vi "RECIPE_NAME_DOWNLOAD.vi"(8 "error in (no error)":errorcluster, 9 "Recipe Names":string[][](array[string]), 10 "appended array":refnum<vi>[](array[refnum])) -> (0 "error out":errorcluster)   [LabVIEW 2017]
panel:
  in  "PRODUCT LIST":string(combo)
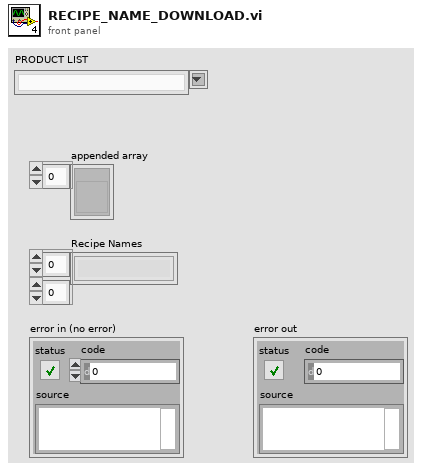
[diagram p1: front panel]
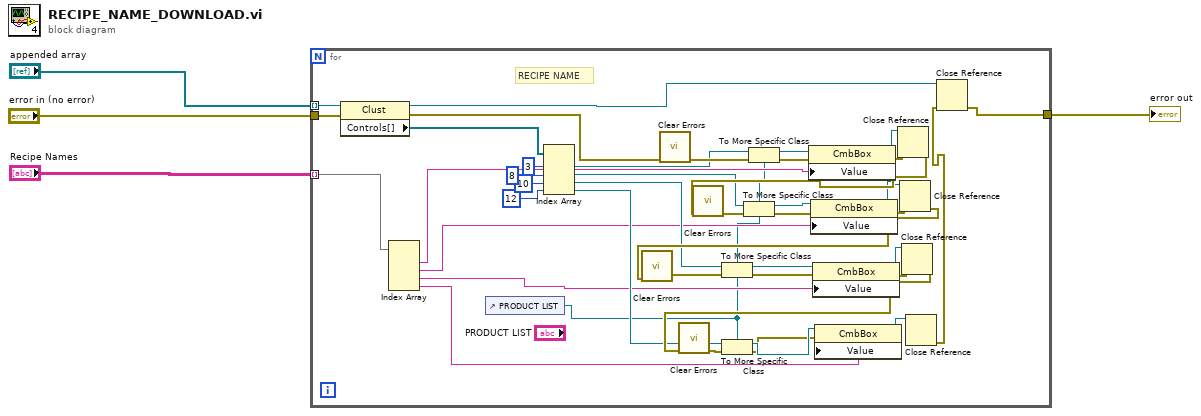
[diagram p0: block diagram]
diagram:
  n1 = for {
    tunnel: [w44] -> w1
    tunnel: "appended array" -> [w47] mode=indexing
    tunnel: "error in (no error)" -> [w46]
    tunnel: "Recipe Names" -> [w27] mode=indexing
    # "RECIPE NAME"
    n2 = property class="Clust"(reference=w47, error in=w46) -> (reference out=w43:refnum<vi>, error out=w45:errorcluster, "Controls[]"=w41:refnum<vi>[])
    n3 = Index Array(array=w27) -> (element #1=w23:string, element #2=w8:string, element #3=w7:string, element #4=w6:string)  [unwired: 4 in]
    n4 = control-ref of="PRODUCT LIST"() -> (w5:refnum<vi>)
    n5 = Index Array(array=w41, index #1=3 ("index"), index #2=8 ("index"), index #3=10 ("index"), index #4=12 ("index")) -> (element #1=w9:refnum<vi>, element #2=w13:refnum<vi>, element #3=w18:refnum<vi>, element #4=w26:refnum<vi>)
    n6 = call <vilib>:"Clear Errors.vi"("error in (no error)"=w45) -> ("error out"=w12:errorcluster)  [unwired: 5 in, 1 out]
    n7 = To More Specific Class(target class=w5, reference=w9, error in=w12) -> (specific class reference=w10:refnum<vi>, error out=w11:errorcluster)
    n8 = property class="CmbBox"(reference=w10, error in=w11, "Value"=w23) -> (reference out=w30:refnum<vi>, error out=w42:errorcluster)
    n9 = Close Reference(reference=w30, error in (no error)=w42) -> (error out=w33:errorcluster)
    n10 = call <vilib>:"Clear Errors.vi"("error in (no error)"=w33) -> ("error out"=w16:errorcluster)  [unwired: 5 in, 1 out]
    n11 = To More Specific Class(target class=w5, reference=w13, error in=w16) -> (specific class reference=w14:refnum<vi>, error out=w15:errorcluster)
    n12 = property class="CmbBox"(reference=w14, error in=w15, "Value"=w8) -> (reference out=w29:refnum<vi>, error out=w36:errorcluster)
    n13 = Close Reference(reference=w29, error in (no error)=w36) -> (error out=w32:errorcluster)
    n14 = call <vilib>:"Clear Errors.vi"("error in (no error)"=w32) -> ("error out"=w19:errorcluster)  [unwired: 5 in, 1 out]
    n15 = To More Specific Class(target class=w5, reference=w18, error in=w19) -> (specific class reference=w17:refnum<vi>, error out=w20:errorcluster)
    n16 = property class="CmbBox"(reference=w17, error in=w20, "Value"=w7) -> (reference out=w28:refnum<vi>, error out=w35:errorcluster)
    n17 = Close Reference(reference=w28, error in (no error)=w35) -> (error out=w31:errorcluster)
    n18 = call <vilib>:"Clear Errors.vi"("error in (no error)"=w31) -> ("error out"=w22:errorcluster)  [unwired: 5 in, 1 out]
    n19 = To More Specific Class(target class=w5, reference=w26, error in=w22) -> (specific class reference=w24:refnum<vi>, error out=w21:errorcluster)
    n20 = property on="Property Node" class="CmbBox"(reference=w24, error in=w21, "Value"=w6) -> (reference out=w25:refnum<vi>)  [unwired: 1 out]
    n21 = Close Reference(reference=w25) -> (error out=w34:errorcluster)  [unwired: 1 in]
    n22 = Close Reference(reference=w43, error in (no error)=w34) -> (error out=w44:errorcluster)
  }
  "error out" <- w1
